vi "UR LabVIEW Interface.vi"() -> ()   [LabVIEW 2016]
uses:
  Classes/Application/Application.lvclass
  Classes/Application/FrontPanelControls.ctl
  Classes/Robot/Universal Robot/Universal Robot.lvclass
  Classes/Robot/UR CB-Series/UR CB-Series.lvclass
  C:/_Code/Development/Sub-Zero Functional Test/standard hardware/Universal Robots/UR LabVIEW Interface/Classes/Robot/Universal Robot/Universal Robot.lvclass
  Classes/Robot/UR E-Series/UR E-Series.lvclass
  Classes/Client Interfaces/Dashboard Server/Dashboard Server.lvclass
  Classes/Client Interfaces/Socket Communication/Socket Communication.lvclass
  Classes/Application/Application Interfaces/Operation Interface/Operation Interface.lvclass
  C:/_Code/Development/Sub-Zero Functional Test/standard hardware/Universal Robots/UR LabVIEW Interface/Classes/Application/Application Interfaces/Application Interface/Application Interface.lvclass
  Classes/Application/Application Interfaces/Command Interface/Command Interface.lvclass
  Classes/Application/Application Interfaces/Program Interface/Program Interface.lvclass
  Classes/Application/Application Interfaces/Socket Auto Connect/Socket Auto Connect.lvclass
  Classes/Application/Application Interfaces/Application Interface/Application Interface.lvclass
panel:
  in  "connect":bool
  in  "status":string
  out "Polyscope Version":string
  in  "abort":bool
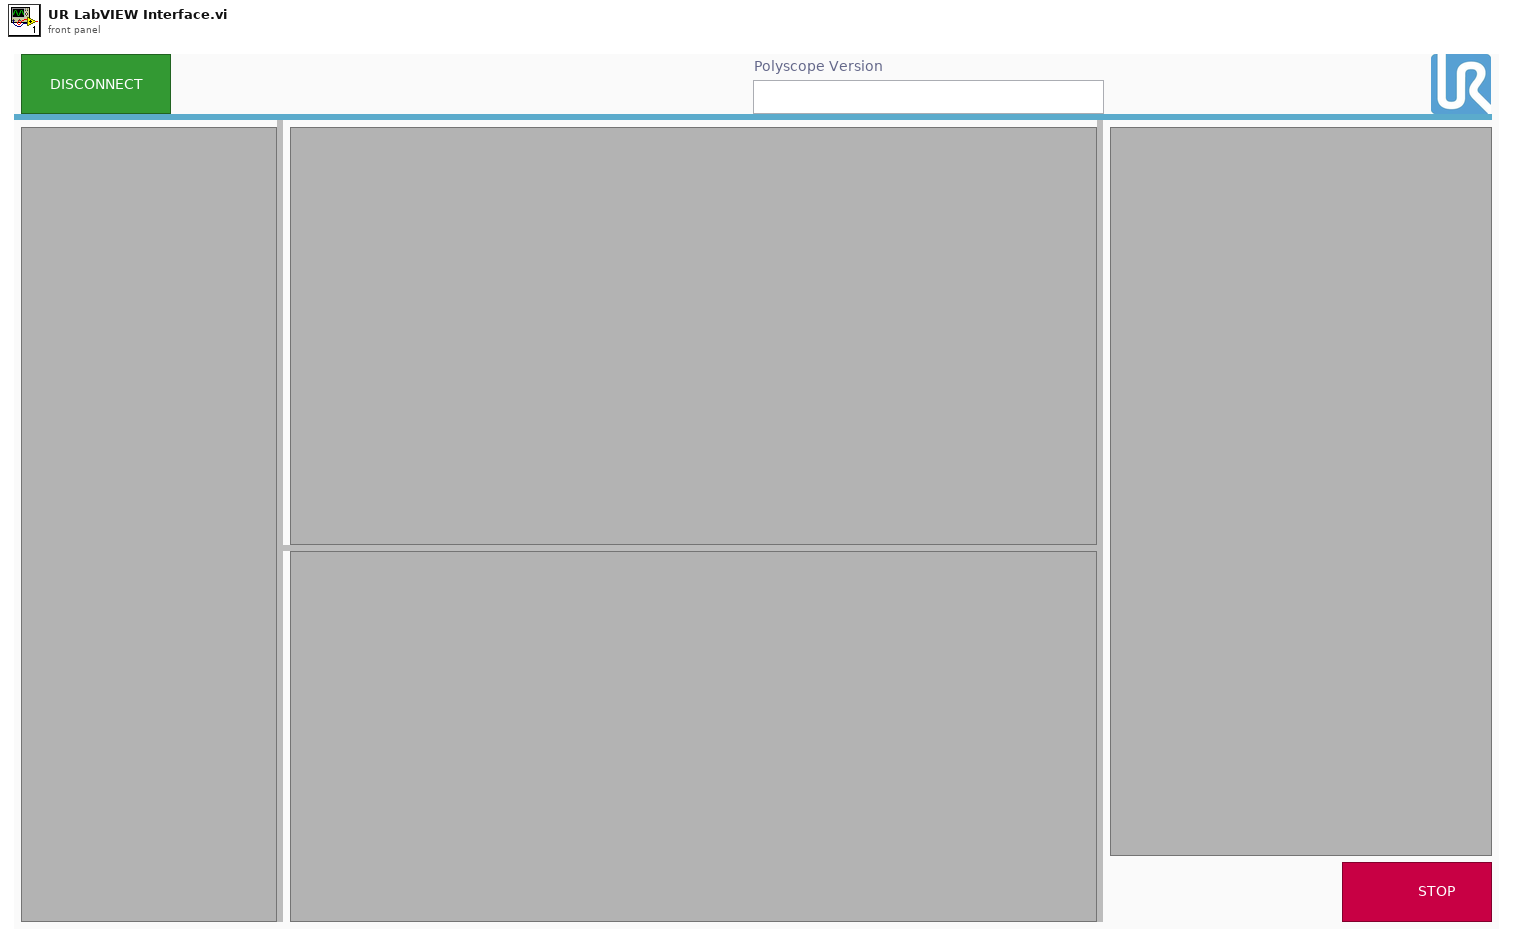
[diagram p1: front panel]
types:
  T1 = typedef "Application.lvclass/FrontPanelControls.ctl" = cluster{"Operation Interface":refnum<vi>, "Program Interface":refnum<vi>, "Command Interface":refnum<vi>, "Socket Interface":refnum<vi>}
  T2 = typedef "Application.lvclass/ApplicationSettings.ctl" = cluster{"Robot IP":string, "Socket Host IP":string, "Robot Type":T3}
  T3 = typedef "Application.lvclass/RobotType.ctl" = enum16{"UR E-Series", "UR CB-Series"}
  T4 = enum32{"invalid app kind", "Development System", "Run Time System", "Student Edition", "Embedded LabVIEW", "Evaluation", "Custom"}
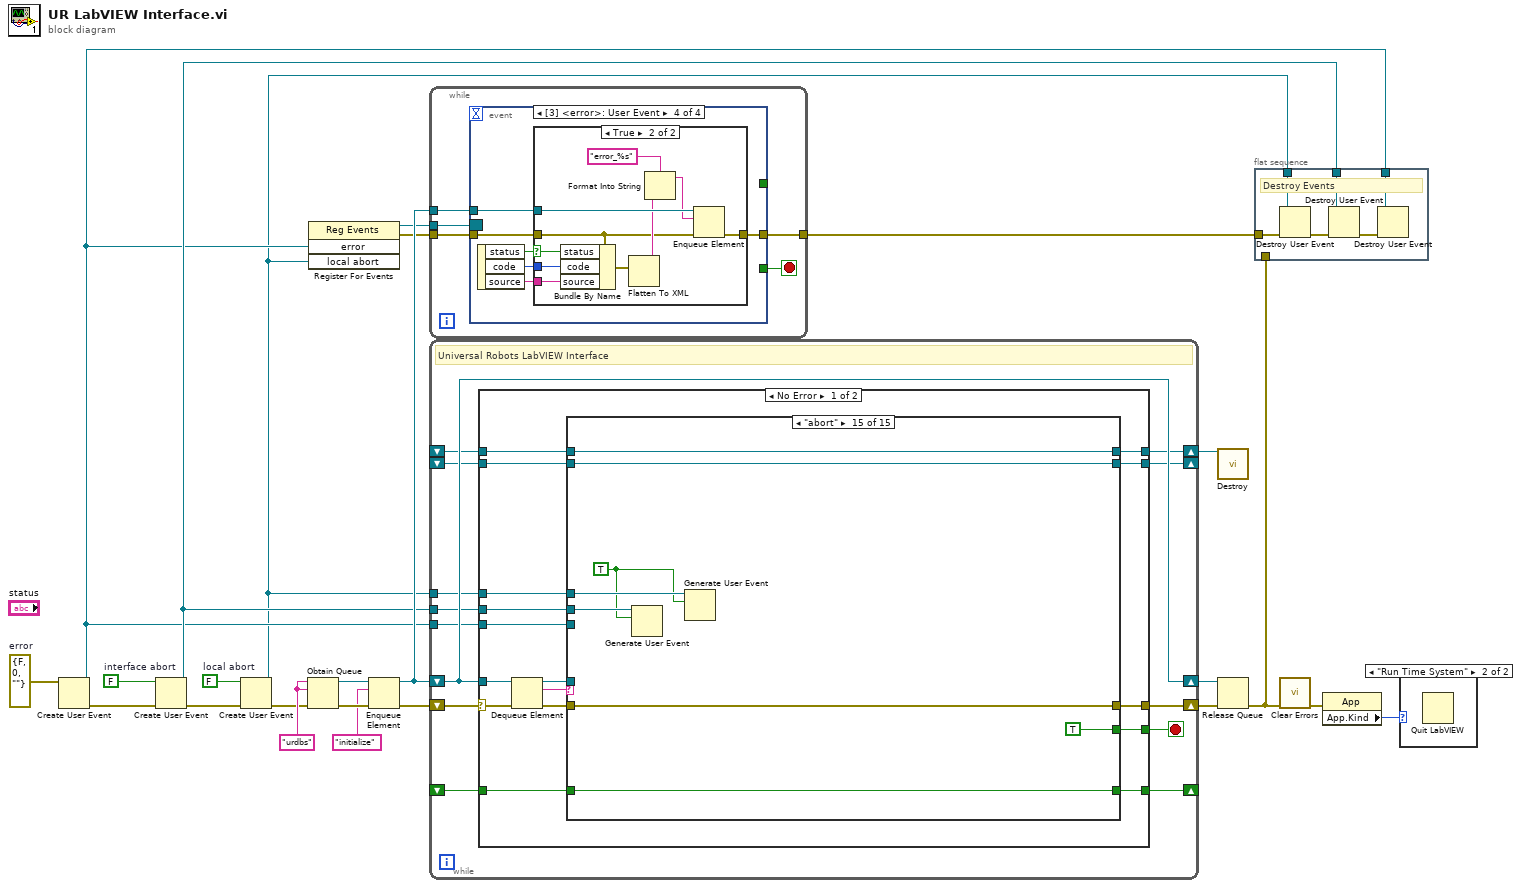
[diagram p0: block diagram]
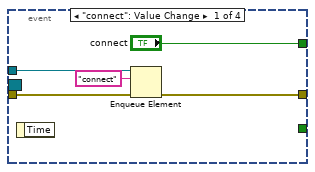
[diagram p3: hidden frame]
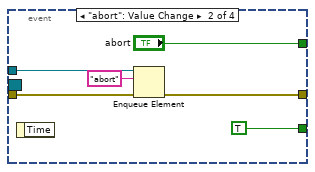
[diagram p4: hidden frame]
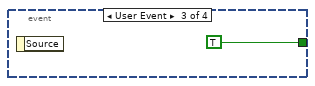
[diagram p5: hidden frame]
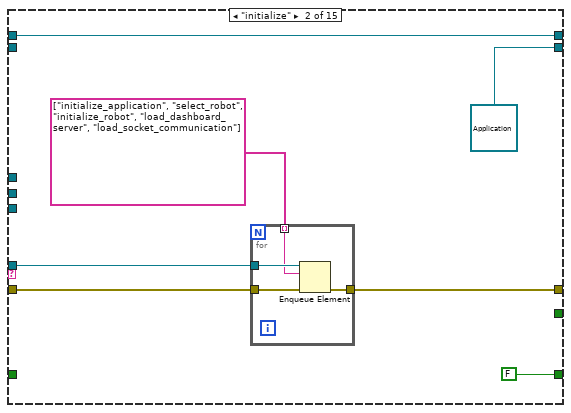
[diagram p8: hidden frame]
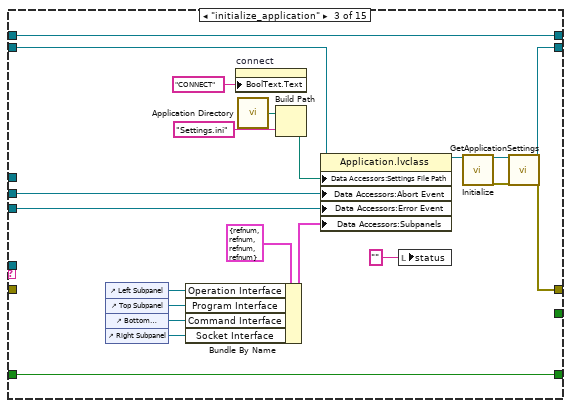
[diagram p9: hidden frame]
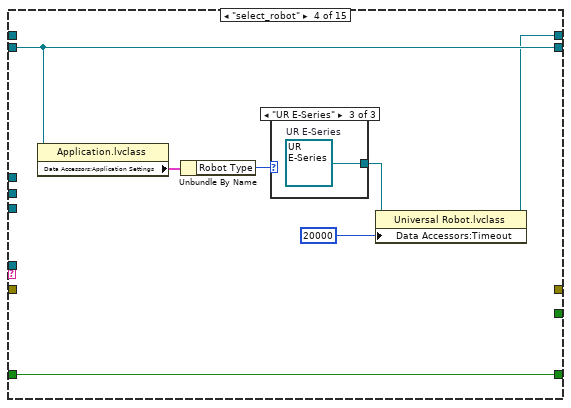
[diagram p10: hidden frame]
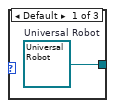
[diagram p11: hidden frame]
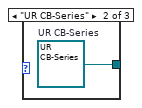
[diagram p12: hidden frame]
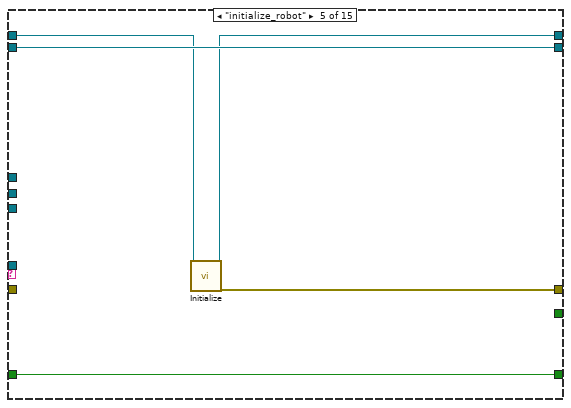
[diagram p13: hidden frame]
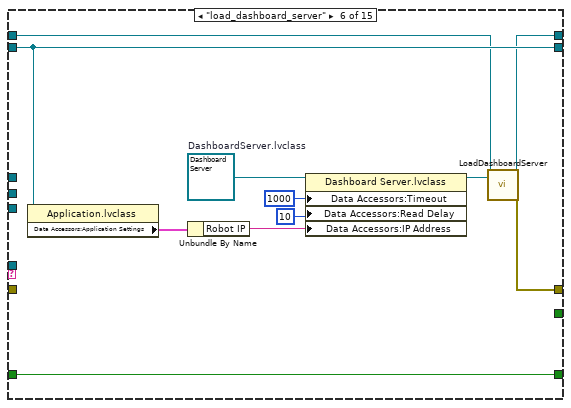
[diagram p14: hidden frame]
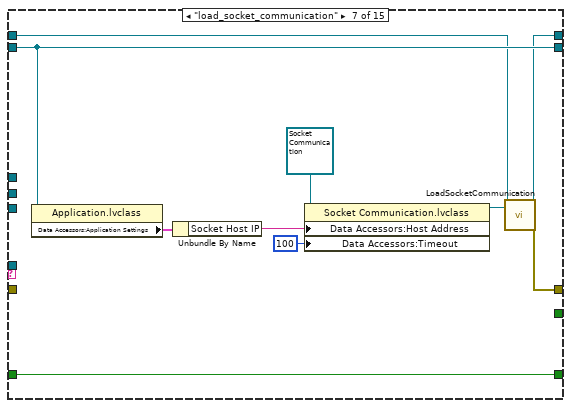
[diagram p15: hidden frame]
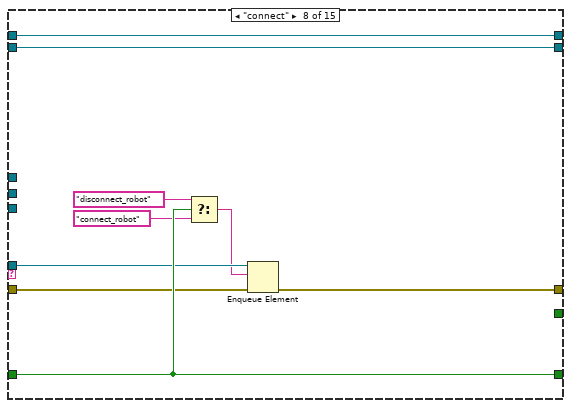
[diagram p16: hidden frame]
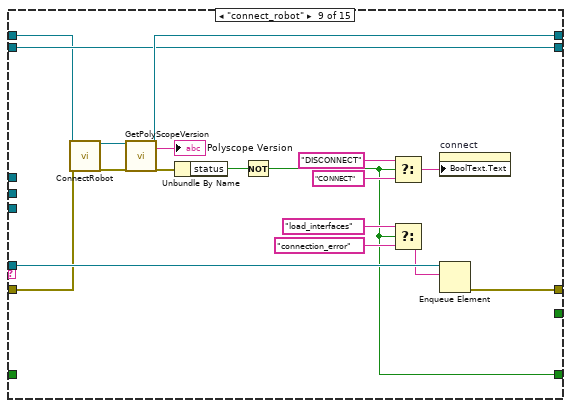
[diagram p17: hidden frame]
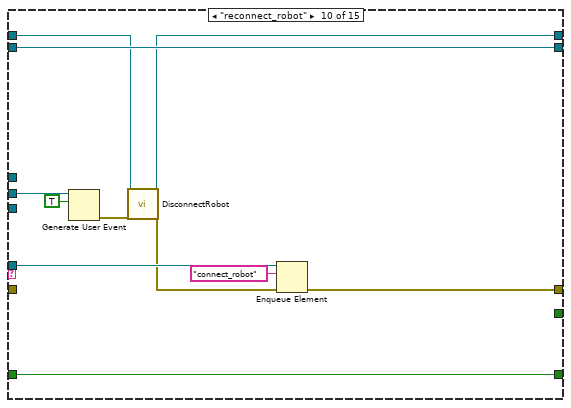
[diagram p18: hidden frame]
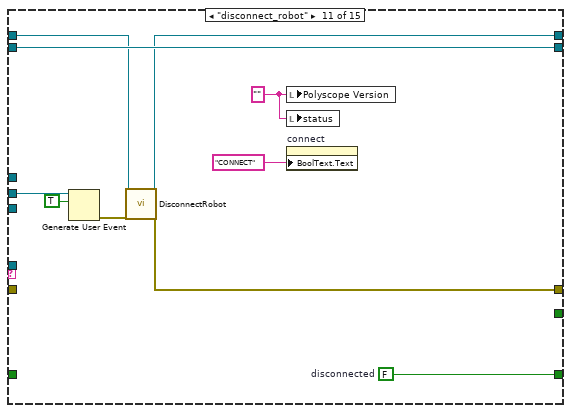
[diagram p19: hidden frame]
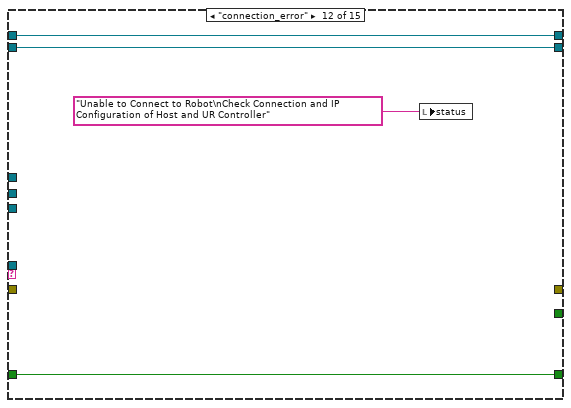
[diagram p20: hidden frame]
diagram:
  w2 = FALSE  # local abort
  w12 = errorcluster {"status"=FALSE, "code"=0, "source"=""}  # error
  w14 = FALSE  # interface abort
  w19 = "urdbs" ("name (unnamed)")
  n1 = Create User Event(user event datatype=w12) -> (user event=w10:refnum<user-event>, error out=w13:errorcluster)  [unwired: 1 in]
  n2 = Create User Event(user event datatype=w14, error in=w13) -> (user event=w11:refnum<user-event>, error out=w4:errorcluster)
  n3 = Create User Event(user event datatype=w2, error in=w4) -> (user event=w1:refnum<user-event>, error out=w3:errorcluster)
  n4 = Obtain Queue(name (unnamed)=w19, element data type=w19, error in (no error)=w3) -> (queue out=w23:refnum<queue>, error out=w24:errorcluster)  [unwired: 2 in, 1 out]
  n5 = register-events(w10, w1) -> (reference out=w5:refnum<event-registration>, error out=w16:errorcluster)  [unwired: 2 in]
  n6 = Enqueue Element(queue=w23, element="initialize", error in (no error)=w24) -> (queue out=w20:refnum<queue>, error out=w21:errorcluster)  [unwired: 1 in, 1 out]
  n7 = while {
    tunnel: w20 -> [w29]
    tunnel: w16 -> [w28]
    tunnel: w5 -> [w27]
    tunnel: [w26] -> w15
    stop <- w25 stop-if-true
    n8 = event shown="[3] <error>: User Event" {
      selector: w27 -> [_ _ _ _]
      dyn-events: _ -> [_ _ _ _]
      timeout: _ -> [_ _ _ _]
      tunnel: w29 -> [w34 w40 _ w45]
      tunnel: w28 -> [w33 w39 _ w42]
      tunnel: [w32 w38 _ w44] -> w26
      tunnel: [_ TRUE TRUE _] -> w25
      tunnel: ["connect" "abort" _ _] -> _
      event "connect": Value Change {
        n9 = event-data() -> ()  [unwired: 1 in, 1 out]
        n10 = Enqueue Element(queue=w34, element="connect", error in (no error)=w33) -> (error out=w32:errorcluster)  [unwired: 1 in, 2 out]
      }
      event "abort": Value Change {
        n11 = event-data() -> ()  [unwired: 1 in, 1 out]
        n12 = Enqueue Element(queue=w40, element="abort", error in (no error)=w39) -> (error out=w38:errorcluster)  [unwired: 1 in, 2 out]
      }
      event User Event {
        n13 = event-data() -> ()  [unwired: 1 in, 1 out]
      }
      event User Event {
        n14 = event-data() -> ("status"=w43:bool, "code"=w47:i32, "source"=w46:string)  [unwired: 1 in]
        n15 = case shown="True" w43 {
          selector: w43 -> [_ w49]
          tunnel: w47 -> [_ w58]
          tunnel: w46 -> [_ w57]
          tunnel: w45 -> [_ w55]
          tunnel: [w48 w54] -> w44
          tunnel: w42 -> [w48 w50]
          frame False {
          }
          frame True {
            n16 = Bundle By Name(cluster=w50, "status"=w49, "code"=w58, "source"=w57) -> (w56:errorcluster)
            n17 = Flatten To XML(anything=w56) -> (xml string=w53:string)
            n18 = Format Into String(format string="error_%s", w53) -> (resulting string=w52:string)  [unwired: 2 in, 1 out]
            n19 = Enqueue Element(queue=w55, element=w52, error in (no error)=w50) -> (error out=w54:errorcluster)  [unwired: 1 in, 2 out]
          }
        }
      }
    }
  }
  n20 = while {
    shift-right: [w69] -> w17
    shift-left: w21 -> [w71]
    shift-right: [w70] -> w18
    shift-left: w20 -> [w70]
    tunnel: w11 -> [w68]
    shift-right: [w66] -> w9
    shift-left: _ -> [w65]
    shift-right: [w64] -> _
    shift-left: _ -> [w63]
    tunnel: w10 -> [w62]
    shift-right: [w61] -> _
    shift-left: _ -> [w60]
    tunnel: w1 -> [w59]
    stop <- w67 stop-if-true
    # "Universal Robots LabVIEW Interface"
    n21 = case shown="No Error" w71 {
      selector: w71 -> [w86 w255]
      tunnel: w70 -> [w87 _]
      tunnel: [w82 _] -> w69
      tunnel: w68 -> [w76 _]
      tunnel: [w81 _] -> w67
      tunnel: [w80 w259] -> w66
      tunnel: w65 -> [w79 w259]
      tunnel: [w78 w258] -> w64
      tunnel: w63 -> [w77 w258]
      tunnel: w62 -> [w75 w256]
      tunnel: [w74 w257] -> w61
      tunnel: w60 -> [w73 w257]
      tunnel: w59 -> [w72 _]
      frame No Error {
        n22 = Dequeue Element(queue=w87, error in (no error)=w86) -> (queue out=w83:refnum<queue>, element=w84:string, error out=w85:errorcluster)  [unwired: 1 in, 1 out]
        n23 = case shown="\"abort\"" w84 {
          selector: w84 -> [_ _ _ _ _ _ _ _ _ _ _ _ _ w239 _]
          tunnel: w85 -> [w91 w98 _ _ _ _ _ w164 w172 _ _ _ w220 w236 w247]
          tunnel: w83 -> [_ w97 _ _ _ _ _ w165 w183 w193 _ _ _ w227 _]
          tunnel: [w91 w96 w105 _ w134 w139 w150 w163 w182 w191 w201 _ w212 _ w247] -> w82
          tunnel: [_ _ _ _ _ _ _ _ _ _ _ _ _ _ TRUE] -> w81
          tunnel: [w90 w92 w123 w125 w135 w140 w151 w168 w186 w194 w205 w211 w216 w242 w253] -> w80
          tunnel: w79 -> [w90 w92 w123 _ w136 w141 w152 w168 w175 w195 w206 w211 w216 w242 w253]
          tunnel: [w89 refnum<class "Application.lvclass"> refnum ("Application.lvclass") w106 w129 w138 w145 w158 w167 w184 w197 w207 w210 w217 w241 w252] -> w78
          tunnel: w77 -> [w89 _ w109 w129 w138 w145 w158 w167 w184 w197 w207 w210 w217 w241 w252]
          tunnel: w76 -> [_ _ w118 _ _ _ _ _ _ w189 w204 _ _ _ w251]
          tunnel: w75 -> [_ _ w117 _ _ _ _ _ _ _ _ _ _ w228 _]
          tunnel: [w88 FALSE ("connected") w115 w130 w137 w146 w159 w166 w169 w196 w198 w209 w221 w240 w250] -> w74
          tunnel: w73 -> [w88 _ w115 w130 w137 w146 w159 w166 _ w196 _ w209 w221 w240 w250]
          tunnel: w72 -> [_ _ _ _ _ _ _ _ _ _ _ _ _ _ w249]
          frame Default {
          }
          frame "initialize" {
            n24 = for {
              tunnel: w98 -> [w102]
              tunnel: w97 -> [w101]
              tunnel: [w100] -> w96
              tunnel: string[] ["initialize_application", "select_robot", "initialize_robot", "load_dashboard_server", "load_socket_communication"] -> [w99] mode=indexing
              n25 = Enqueue Element(queue=w101, element=w99, error in (no error)=w102) -> (error out=w100:errorcluster)  [unwired: 1 in, 2 out]
            }
          }
          frame "initialize_application" {
            n26 = control-ref of="Left Subpanel"() -> (w121:refnum<vi>)
            n27 = control-ref of="Top Subpanel"() -> (w120:refnum<vi>)
            n28 = control-ref of="Bottom Subpanel"() -> (w119:refnum<vi>)
            n29 = control-ref of="Right Subpanel"() -> (w103:refnum<vi>)
            n30 = Bundle By Name(cluster=T1 {"Operation Interface"=refnum, "Program Interface"=refnum, "Command Interface"=refnum, "Socket Interface"=refnum} ("frontPanelControls"), "Operation Interface"=w121, "Program Interface"=w120, "Command Interface"=w119, "Socket Interface"=w103) -> (w116:T1)
            n31 = property on="connect" class="Bool"("BoolText.Text"="CONNECT" ("Boolean Text.Text")) -> ()  [unwired: 2 in, 2 out]
            n32 = call <vilib>:"Application Directory.vi"() -> ("Application Directory"=w111:path)
            n33 = Build Path(base path=w111, name or relative path="Settings.ini") -> (appended path=w112:path)
            n34 = property class="Application.lvclass"(reference=w109, "Data Accessors:Settings File Path"=w112, "Data Accessors:Abort Event"=w118, "Data Accessors:Error Event"=w117, "Data Accessors:Subpanels"=w116) -> (reference out=w113:refnum<class "Application.lvclass">)  [unwired: 1 in, 1 out]
            n35 = local write "status"("" ("status")) -> ()
            n36 = call-dynamic "Initialize.vi"("Application in"=w113) -> ("Application out"=w108:refnum<class "Application.lvclass">, "error out"=w107:errorcluster)  [unwired: 17 in]
            n37 = call-dynamic "GetApplicationSettings.vi"("Application in"=w108, "error in (no error)"=w107) -> ("Application out"=w106:refnum<class "Application.lvclass">, "error out"=w105:errorcluster)  [unwired: 16 in]
          }
          frame "select_robot" {
            n38 = property class="Application.lvclass"(reference=w129) -> ("Data Accessors:Application Settings"=w128:T2)  [unwired: 1 in, 2 out]
            n39 = Unbundle By Name(w128) -> ("Robot Type"=w127:T3)
            n40 = case shown="\"UR E-Series\"" w127 {
              tunnel: [w131 w132 w133] -> w126
              frame Default {
                w131 = refnum<class "Universal Robot.lvclass"> refnum  # Universal Robot
              }
              frame "UR CB-Series" {
                w132 = refnum<class "UR CB-Series.lvclass"> refnum  # UR CB-Series
              }
              frame "UR E-Series" {
                w133 = refnum<class "UR E-Series.lvclass"> refnum  # UR E-Series
              }
            }
            n41 = property class="Universal Robot.lvclass"(reference=w126, "Data Accessors:Timeout"=u32 20000 ("Timeout")) -> (reference out=w125:refnum<class "Universal Robot.lvclass">)  [unwired: 1 in, 1 out]
          }
          frame "initialize_robot" {
            n42 = call-dynamic "Initialize.vi"("Universal Robot in"=w136) -> ("Universal Robot out"=w135:refnum<class "Universal Robot.lvclass">, "error out"=w134:errorcluster)  [unwired: 17 in]
          }
          frame "load_dashboard_server" {
            w149 = refnum<class "Dashboard Server.lvclass"> refnum  # DashboardServer.lvclass
            n43 = property class="Application.lvclass"(reference=w145) -> ("Data Accessors:Application Settings"=w144:T2)  [unwired: 1 in, 2 out]
            n44 = Unbundle By Name(w144) -> ("Robot IP"=w143:string)
            n45 = property class="Dashboard Server.lvclass"(reference=w149, "Data Accessors:Timeout"=1000 ("timeout"), "Data Accessors:Read Delay"=u32 10 ("readDelay"), "Data Accessors:IP Address"=w143) -> (reference out=w142:refnum<class "Dashboard Server.lvclass">)  [unwired: 1 in, 1 out]
            n46 = call-dynamic "LoadDashboardServer.vi"("Universal Robot in"=w141, "DashboardServer"=w142) -> ("Universal Robot out"=w140:refnum<class "Universal Robot.lvclass">, "error out"=w139:errorcluster)  [unwired: 16 in]
          }
          frame "load_socket_communication" {
            n47 = property class="Application.lvclass"(reference=w158) -> ("Data Accessors:Application Settings"=w157:T2)  [unwired: 1 in, 2 out]
            n48 = Unbundle By Name(w157) -> ("Socket Host IP"=w156:string)
            n49 = property class="Socket Communication.lvclass"(reference=refnum<class "Socket Communication.lvclass"> refnum ("TCP Socket.lvclass"), "Data Accessors:Host Address"=w156, "Data Accessors:Timeout"=100 ("Timeout")) -> (reference out=w153:refnum<class "Socket Communication.lvclass">)  [unwired: 1 in, 1 out]
            n50 = call-dynamic "LoadSocketCommunication.vi"("Universal Robot in"=w152, "Socket Communication"=w153) -> ("Universal Robot out"=w151:refnum<class "Universal Robot.lvclass">, "error out"=w150:errorcluster)  [unwired: 16 in]
          }
          frame "connect" {
            n51 = Select(t="disconnect_robot", s=w166, f="connect_robot") -> (s? t:f=w160:string)
            n52 = Enqueue Element(queue=w165, element=w160, error in (no error)=w164) -> (error out=w163:errorcluster)  [unwired: 1 in, 2 out]
          }
          frame "connect_robot" {
            n53 = call-dynamic "ConnectRobot.vi"("Universal Robot.lvclass in"=w175, "error in (no error)"=w172) -> ("Universal Robot.lvclass out"=w174:refnum<class "Universal Robot.lvclass">, "error out"=w173:errorcluster)  [unwired: 16 in]
            n54 = call-dynamic "GetPolyScopeVersion.vi"("Universal Robot.lvclass in"=w174, "error in (no error)"=w173) -> ("Universal Robot.lvclass out"=w186:refnum<class "Universal Robot.lvclass">, "polyscopeVersion"=→"Polyscope Version":string, "error out"=w171:errorcluster)  [unwired: 15 in]
            n55 = Unbundle By Name(w171) -> ("status"=w170:bool)
            n56 = Not(x=w170) -> (.not. x?=w169:bool)
            n57 = Select(t="DISCONNECT" ("Boolean Text.Text"), s=w169, f="CONNECT" ("Boolean Text.Text")) -> (s? t:f=w176:string)
            n58 = Select(t="load_interfaces", s=w169, f="connection_error") -> (s? t:f=w180:string)
            n59 = property on="connect" class="Bool"("BoolText.Text"=w176) -> ()  [unwired: 2 in, 2 out]
            n60 = Enqueue Element(queue=w183, element=w180) -> (error out=w182:errorcluster)  [unwired: 2 in, 2 out]
          }
          frame "reconnect_robot" {
            n61 = Generate User Event(user event=w189, event data cluster=TRUE ("event data")) -> (error out=w187:errorcluster)  [unwired: 2 in, 1 out]
            n62 = call-dynamic "DisconnectRobot.vi"("Universal Robot.lvclass in"=w195, "error in (no error)"=w187) -> ("Universal Robot.lvclass out"=w194:refnum<class "Universal Robot.lvclass">, "error out"=w192:errorcluster)  [unwired: 16 in]
            n63 = Enqueue Element(queue=w193, element="connect_robot", error in (no error)=w192) -> (error out=w191:errorcluster)  [unwired: 1 in, 2 out]
          }
          frame "disconnect_robot" {
            w198 = FALSE  # disconnected
            w200 = "" ("polyscopeVersion")
            n64 = Generate User Event(user event=w204, event data cluster=TRUE ("event data")) -> (error out=w202:errorcluster)  [unwired: 2 in, 1 out]
            n65 = call-dynamic "DisconnectRobot.vi"("Universal Robot.lvclass in"=w206, "error in (no error)"=w202) -> ("Universal Robot.lvclass out"=w205:refnum<class "Universal Robot.lvclass">, "error out"=w201:errorcluster)  [unwired: 16 in]
            n66 = local write "Polyscope Version"(w200) -> ()
            n67 = local write "status"(w200) -> ()
            n68 = property on="connect" class="Bool"("BoolText.Text"="CONNECT" ("Boolean Text.Text")) -> ()  [unwired: 2 in, 2 out]
          }
          frame "connection_error" {
            n69 = local write "status"("Unable to Connect to Robot\nCheck Connection and IP Configuration of Host and UR Controller" ("status")) -> ()
          }
          frame "load_interfaces" {
            n70 = Build Array(refnum<class "Operation Interface.lvclass"> refnum ("Operation Interface.lvclass"), refnum<class "Command Interface.lvclass"> refnum ("Command Interface.lvclass"), refnum<class "Program Interface.lvclass"> refnum ("Program Interface.lvclass"), refnum<class "Socket Auto Connect.lvclass"> refnum ("Auto Connect TCP Socket Viewer.lvclass")) -> (w218:refnum<class "Application Interface.lvclass">[])
            n71 = for {
              tunnel: w220 -> [w226]
              tunnel: w218 -> [w225] mode=indexing
              tunnel: w217 -> [w224]
              tunnel: w216 -> [w223]
              tunnel: [w222] -> w212
              n72 = call "LoadInterface.vi"("Application Interface in"=w225, "application"=w224, "universalRobot"=w223, "error in (no error)"=w226) -> ("error out"=w222:errorcluster)  [unwired: 14 in, 1 out]
            }
          }
          frame "error_".."error_~" {
            n73 = Match Pattern(string=w239, regular expression="_") -> (after substring=w237:string)  [unwired: 1 in, 3 out]
            n74 = Unflatten From XML(xml string=w237, type=w236) -> (value=w235:errorcluster)  [unwired: 1 in, 1 out]
            n75 = Unbundle By Name(w235) -> ("source"=w234:string)
            n76 = Format Into String(format string="Error Occured!\n\n%s", w234) -> (resulting string=w230:string)  [unwired: 2 in, 1 out]
            n77 = Two Button Dialog(message=w230, 1:"Abort" ("F button name (\"Cancel\")"), 2:"Clear" ("T button name (\"OK\")")) -> (T button?=w229:bool)
            n78 = case shown="False" w229 {
              tunnel: w228 -> [_ w246]
              tunnel: w227 -> [w244 _]
              frame False {
                n79 = Enqueue Element At Opposite End(queue=w244, element="abort") -> ()  [unwired: 2 in, 3 out]
              }
              frame True {
                n80 = Generate User Event(user event=w246, event data cluster=errorcluster {"status"=FALSE, "code"=0, "source"=""} ("event data")) -> ()  [unwired: 2 in, 2 out]
              }
            }
          }
          frame "abort" {
            w248 = TRUE ("event data")
            n81 = Generate User Event(user event=w251, event data cluster=w248) -> ()  [unwired: 2 in, 2 out]
            n82 = Generate User Event(user event=w249, event data cluster=w248) -> ()  [unwired: 2 in, 2 out]
          }
        }
      }
      frame Error {
        n83 = Generate User Event(user event=w256, event data cluster=w255) -> ()  [unwired: 2 in, 2 out]
      }
    }
  }
  n84 = call-dynamic "Destroy.vi"("Universal Robot in"=w9) -> ()  [unwired: 17 in, 2 out]
  n85 = Release Queue(queue=w18, error in (no error)=w17) -> (error out=w6:errorcluster)  [unwired: 1 in, 2 out]
  n86 = flat-sequence {
    tunnel: w15 -> [w262]
    tunnel: w11 -> [w265]
    tunnel: w10 -> [w263]
    tunnel: w6 -> [_]
    tunnel: w1 -> [w260]
    frame #0 {
      # "Destroy Events"
      n87 = Destroy User Event(user event=w260, error in=w262) -> (error out=w261:errorcluster)
      n88 = Destroy User Event(user event=w265, error in=w261) -> (error out=w264:errorcluster)
      n89 = Destroy User Event(user event=w263, error in=w264) -> ()  [unwired: 1 out]
    }
  }
  n90 = call <vilib>:"Clear Errors.vi"("error in (no error)"=w6) -> ("error out"=w8:errorcluster)  [unwired: 5 in, 1 out]
  n91 = property class="App"(error in=w8) -> ("App.Kind"=w7:T4)  [unwired: 1 in, 2 out]
  n92 = case shown="\"Run Time System\"" w7 {
    frame Default {
    }
    frame "Run Time System" {
      n93 = Quit LabVIEW() -> ()  [unwired: 1 in]
    }
  }
